vi "dll good.vi"() -> ()   [LabVIEW 2017]
uses:
  cuda_QI_v2.dll
panel:
  out "c 2":i32
  in  "c":i32
  in  "b":i32
  in  "a":i32
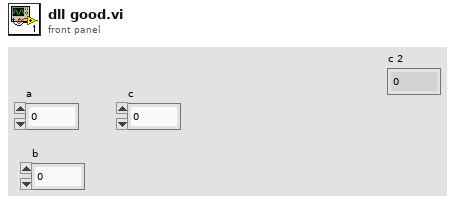
[diagram p1: front panel]
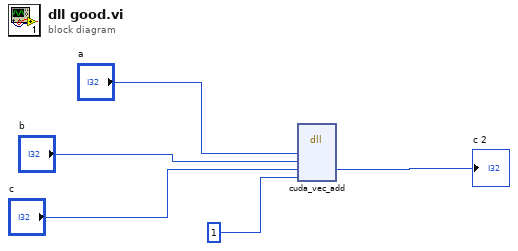
[diagram p0: block diagram]
diagram:
  n1 = dll-call lib="C:/Users/user/Documents/Visual Studio 2015/Projects/cuda_QI_v2/x64/Release/cuda_QI_v2.dll" fn="cuda_vec_add"("a"="a", "b"="b", "c"="c", "n"=1) -> ("c"=→"c 2":i32)  [unwired: 7 in, 2 out]
